vi "Get-Set Color Array.vi"(6 "Clear All":bool, 8 "Get (F)/Set (T)":bool, 10 "Color Array (in)":u32[](array[numeric]), 11 "Color List Name":string) -> (0 "Found?":bool, 1 "# Colors":i32, 2 "Color Array (out)":u32[](array[numeric]), 3 "Color List Name (dup)":string, 4 "Color Arrays (out)":cluster{"Color Array":u32[]}[](array[cluster]), 5 "Color List Name (out)":string[](array[string]))   [LabVIEW 2021]
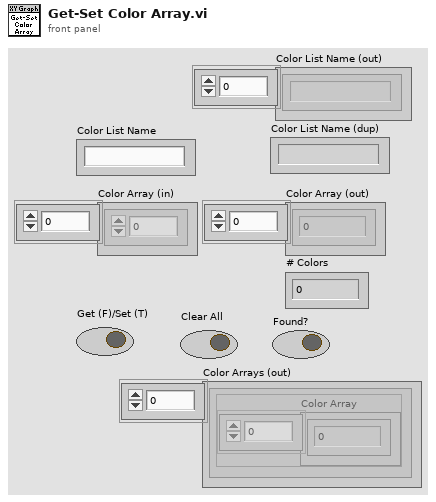
[diagram p1: front panel]
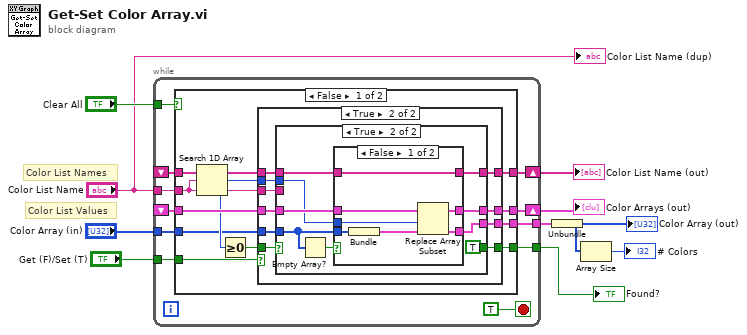
[diagram p0: block diagram]
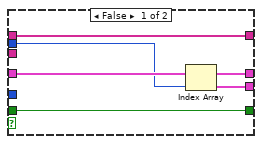
[diagram p2: hidden frame]
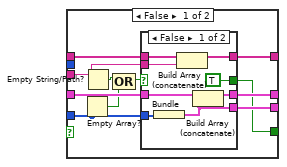
[diagram p3: hidden frame]
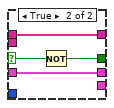
[diagram p4: hidden frame]
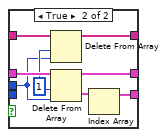
[diagram p5: hidden frame]
diagram:
  # "Color List Values"
  # "Color List Names"
  n1 = while {
    shift-right: [w19] -> w2
    shift-left: _ -> [w17]
    shift-right: [w18] -> w1
    shift-left: _ -> [w16]
    tunnel: "Clear All" -> [w20]
    tunnel: "Get (F)/Set (T)" -> [w15]
    tunnel: "Color List Name" -> [w14]
    tunnel: [w13] -> w8
    tunnel: [w12] -> w7
    tunnel: "Color Array (in)" -> [w11]
    stop <- TRUE stop-if-true
    n2 = case shown="False" w20 {
      tunnel: [w26 _] -> w19
      tunnel: [w27 _] -> w18
      tunnel: w17 -> [w30 _]
      tunnel: w16 -> [w29 _]
      tunnel: w15 -> [w32 _]
      tunnel: w14 -> [w31 _]
      tunnel: [w22 _] -> w13
      tunnel: [w28 _] -> w12
      tunnel: w11 -> [w23 _]
      frame False {
        n3 = Search 1D Array(1D array=w30, element=w31) -> (index of element=w25:i32)  [unwired: 1 in]
        n4 = Greater Or Equal To 0?(x=w25) -> (x >= 0?=w24:bool)
        n5 = case shown="True" w32 {
          tunnel: w31 -> [_ w39]
          tunnel: w30 -> [w35 w46]
          tunnel: w29 -> [w36 w45]
          tunnel: [w37 w40] -> w28
          tunnel: [w36 w42] -> w27
          tunnel: [w35 w41] -> w26
          tunnel: w25 -> [w34 w43]
          tunnel: w24 -> [w33 w47]
          tunnel: w23 -> [_ w44]
          tunnel: [w33 w38] -> w22
          frame False {
            n6 = Index Array(array=w36, index=w34) -> (element=w37:cluster{"Color Array (in)":u32[]})
          }
          frame True {
            n7 = case shown="True" w47 {
              tunnel: w46 -> [w58 w73]
              tunnel: w45 -> [w54 w79]
              tunnel: w44 -> [w51 w75]
              tunnel: w43 -> [_ w78]
              tunnel: [w50 w77] -> w42
              tunnel: [w57 w72] -> w41
              tunnel: [w49 w76] -> w40
              tunnel: w39 -> [w56 _]
              tunnel: [w48 TRUE] -> w38
              frame False {
                n8 = Empty Array?(array=w51) -> (empty?=w52:bool)
                n9 = Empty String/Path?(string/path=w56) -> (empty?=w55:bool)
                n10 = Compound Arithmetic op=OR(w55, w52) -> (w53:bool)
                n11 = case shown="False" w53 {
                  selector: w53 -> [_ w68]
                  tunnel: w58 -> [w66 w70]
                  tunnel: [w65 w70] -> w57
                  tunnel: w56 -> [w64 _]
                  tunnel: w54 -> [w63 w69]
                  tunnel: w51 -> [w62 _]
                  tunnel: [w61 w69] -> w50
                  tunnel: [w60 _] -> w49
                  tunnel: [TRUE w67] -> w48
                  frame False {
                    n12 = Bundle("Color Array (in)"=w62) -> (w60:cluster{"Color Array (in)":u32[]})  [unwired: 1 in]
                    n13 = Build Array (concatenate)(w66, w64) -> (w65:string[])
                    n14 = Build Array (concatenate)(w63, w60) -> (w61:cluster{"Color Array (in)":u32[]}[])
                  }
                  frame True {
                    n15 = Not(x=w68) -> (.not. x?=w67:bool)
                  }
                }
              }
              frame True {
                n16 = Empty Array?(array=w75) -> (empty?=w74:bool)
                n17 = case shown="False" w74 {
                  tunnel: w79 -> [w85 w93]
                  tunnel: w78 -> [w84 w88]
                  tunnel: [w83 w92] -> w77
                  tunnel: [w82 w86] -> w76
                  tunnel: w75 -> [w81 _]
                  tunnel: w73 -> [w80 w91]
                  tunnel: [w80 w90] -> w72
                  frame False {
                    n18 = Bundle("Color Array (in)"=w81) -> (w82:cluster{"Color Array (in)":u32[]})  [unwired: 1 in]
                    n19 = Replace Array Subset(array=w85, new element=w82, index=w84) -> (w83:cluster{"Color Array (in)":u32[]}[])
                  }
                  frame True {
                    w89 = 1 ("length")
                    n20 = Delete From Array(array=w91, length=w89, index=w88) -> (array with subset deleted=w90:string[])  [unwired: 1 out]
                    n21 = Delete From Array(array=w93, length=w89, index=w88) -> (deleted portion=w87:cluster{"Color Array (in)":u32[]}[], array with subset deleted=w92:cluster{"Color Array (in)":u32[]}[])
                    n22 = Index Array(array=w87) -> (element=w86:cluster{"Color Array (in)":u32[]})  [unwired: 1 in]
                  }
                }
              }
            }
          }
        }
      }
      frame True {
      }
    }
  }
  "Found?" <- w8
  "Color List Name (out)" <- w2
  "Color Arrays (out)" <- w1
  n23 = Unbundle(w7) -> ("Color Array (in)"=w4:u32[])
  "Color Array (out)" <- w4
  n24 = Array Size(array=w4) -> (size(s)=→"# Colors":i32)
  "Color List Name (dup)" <- "Color List Name"
